vi "CH1_Tx_TCPIP.vi"() -> ()   [LabVIEW 2018]
uses:
  RxTx/RxTx.lvclass
  TCPIP/TCPIP.lvclass
  TCPIP/TCPIP.lvclass/TCPIP.ctl
panel:
  in  "TCPIP in":refnum<class "TCPIP.lvclass">
  in  "Channel:":u16=1
  in  "RxTx.lvclass":refnum<class "RxTx.lvclass">
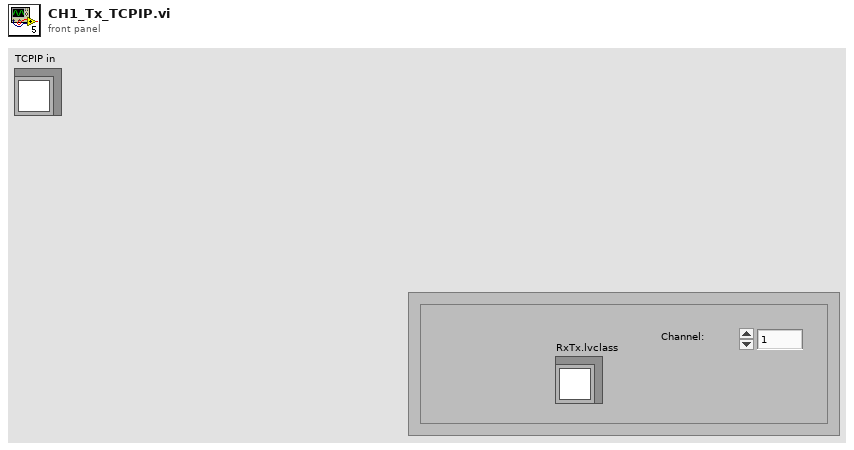
[diagram p1: front panel]
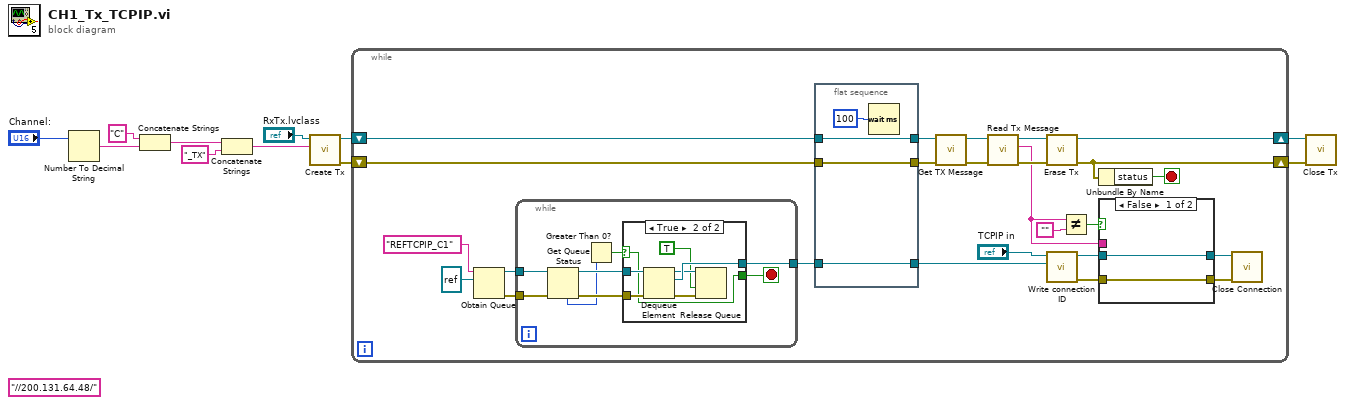
[diagram p0: block diagram]
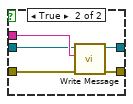
[diagram p2: hidden frame]
diagram:
  (unwired) "//200.131.64.48/" ("Reader Name")
  n1 = Number To Decimal String(number="Channel:") -> (decimal integer string=w5:string)  [unwired: 1 in]
  n2 = Concatenate Strings("C", w5) -> (w2:string)
  n3 = Concatenate Strings(w2, "_TX" ("Reader Name")) -> (w3:string)
  n4 = call "Create Tx.vi"("Writer Name"=w3, "RxTx in"="RxTx.lvclass") -> ("error out"=w10:errorcluster, "RxTx out"=w11:refnum<class "RxTx.lvclass">)  [unwired: 8 in]
  n5 = while {
    shift-right: [w31] -> w8
    shift-left: w10 -> [w13]
    shift-right: [w33] -> w9
    shift-left: w11 -> [w14]
    stop <- w28 stop-if-true
    n6 = Obtain Queue(name (unnamed)="REFTCPIP_C1", element data type=refnum<k5> refnum ("connection ID out")) -> (queue out=w22:refnum<queue>, error out=w21:errorcluster)  [unwired: 3 in, 1 out]
    n7 = while {
      tunnel: w22 -> [w50]
      tunnel: w21 -> [w49]
      tunnel: [w48] -> w17
      stop <- w51 stop-if-true
      n8 = Get Queue Status(queue=w50, error in (no error)=w49) -> (queue out=w55:refnum<queue>, error out=w54:errorcluster, # elements in queue=w52:i32)  [unwired: 1 in, 5 out]
      n9 = Greater Than 0?(x=w52) -> (x > 0?=w53:bool)
      n10 = case shown="True" w53 {
        selector: w53 -> [w56 w61]
        tunnel: w55 -> [_ w63]
        tunnel: w54 -> [_ w62]
        tunnel: [w56 w61] -> w51
        tunnel: [_ w60] -> w48
        frame False {
        }
        frame True {
          n11 = Dequeue Element(queue=w63, error in (no error)=w62) -> (queue out=w59:refnum<queue>, element=w60:refnum<k5>, error out=w58:errorcluster)  [unwired: 1 in, 1 out]
          n12 = Release Queue(queue=w59, force destroy? (F)=TRUE, error in (no error)=w58) -> ()  [unwired: 3 out]
        }
      }
    }
    n13 = flat-sequence {
      tunnel: w17 -> [w39]
      tunnel: [w39] -> w16
      tunnel: [w38] -> w15
      tunnel: w14 -> [w38]
      tunnel: w13 -> [w37]
      tunnel: [w37] -> w12
      frame #0 {
        n14 = Wait (ms)(milliseconds to wait=u32 100) -> ()  [unwired: 1 out]
      }
    }
    n15 = call "Get TX Message.vi"("error in (no error)"=w12, "RxTx in"=w15) -> ("error out"=w36:errorcluster, "RxTx out"=w30:refnum<class "RxTx.lvclass">)  [unwired: 8 in]
    n16 = call "Read Tx Message.vi"("error in (no error)"=w36, "RxTx in"=w30) -> ("error out"=w32:errorcluster, "Tx Message"=w29:string, "RxTx out"=w34:refnum<class "RxTx.lvclass">)  [unwired: 7 in]
    n17 = call "Erase Tx.vi"("error in (no error)"=w32, "RxTx in"=w34) -> ("error out"=w31:errorcluster, "RxTx out"=w33:refnum<class "RxTx.lvclass">)  [unwired: 8 in]
    n18 = call "Write connection ID.vi"("connection ID"=w16, "TCPIP in"="TCPIP in") -> ("error out"=w26:errorcluster, "TCPIP out"=w27:refnum<class "TCPIP.lvclass">)  [unwired: 8 in]
    n19 = Not Equal?(x=w29, y="") -> (x != y?=w18:bool)
    n20 = Unbundle By Name(w31) -> ("status"=w28:bool)
    n21 = case shown="False" w18 {
      tunnel: w29 -> [_ w47]
      tunnel: w27 -> [w42 w46]
      tunnel: w26 -> [w41 w45]
      tunnel: [w42 w44] -> w25
      tunnel: [w41 w43] -> w24
      frame False {
      }
      frame True {
        n22 = call "Write Message.vi"("error in (no error)"=w45, "Message"=w47, "TCPIP in"=w46) -> ("error out"=w43:errorcluster, "TCPIP out"=w44:refnum<class "TCPIP.lvclass">)  [unwired: 7 in]
      }
    }
    n23 = call "Close Connection.vi"("error in (no error)"=w24, "TCPIP in"=w25) -> ()  [unwired: 8 in, 2 out]
  }
  n24 = call "Close Tx.vi"("error in (no error)"=w8, "RxTx in"=w9) -> ()  [unwired: 8 in, 2 out]
